vi "Read From VS Parameter FIFO.vi"(8 "Error In":errorcluster, 11 "Async State Vars":T1) -> (0 "Error Out":errorcluster, 1 "Parameter FIFO empty?":bool, 3 "Async State Vars out":T1)   [LabVIEW 2014, in "Waveform-Processing-Custom-Device Engine.lvlib"]
uses:
  Waveform-Processing-Custom-Device Engine.lvlib
  Types/Async State Vars.ctl
  Types/Async FIFOs.ctl
  <vilib>/NI Veristand/Custom Device Waveform API/Single Waveform Read (DBL)/Single Waveform Read (DBL).lvclass
  <vilib>/NI Veristand/Custom Device Waveform API/Single Waveform Write (DBL)/Single Waveform Write (DBL).lvclass
  <vilib>/NI Veristand/Custom Device API/Waveform Data Reference.ctl
  <vilib>/NI Veristand/Custom Device API/Custom Device API.lvlib
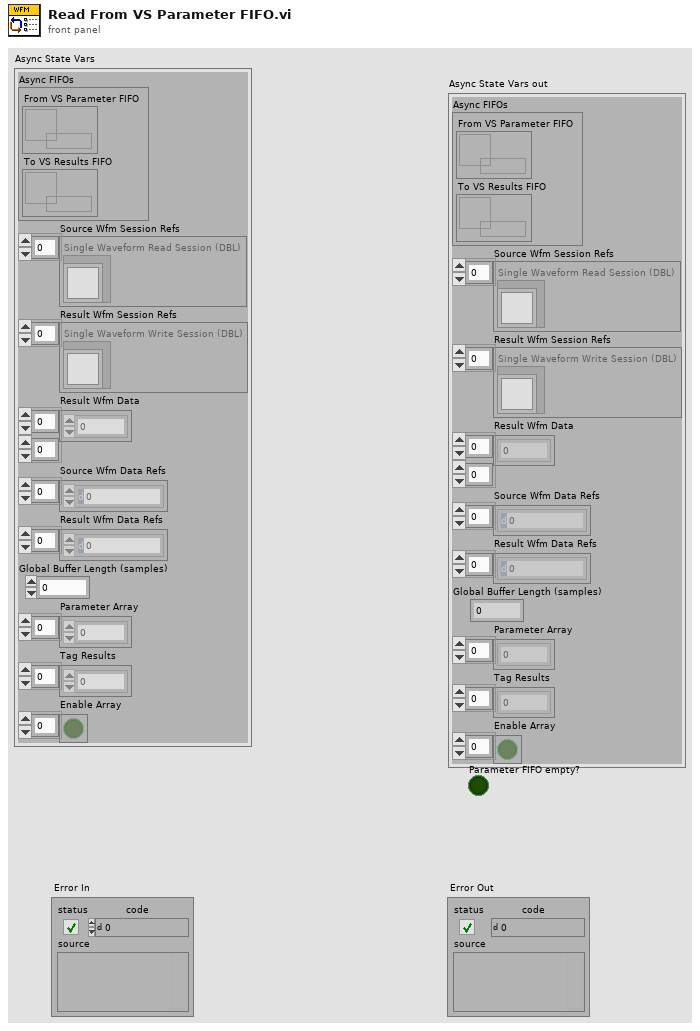
[diagram p1: front panel]
types:
  T1 = typedef "Waveform-Processing-Custom-Device Engine.lvlib/Async State Vars.ctl" = cluster{"Async FIFOs":T2, "Source Wfm Session Refs":refnum<class "Single Waveform Read (DBL).lvclass">[], "Result Wfm Session Refs":refnum<class "Single Waveform Write (DBL).lvclass">[], "Result Wfm Data":dbl[][], "Source Wfm Data Refs":T3[], "Result Wfm Data Refs":T3[], "Global Buffer Length (samples)":dbl, "Parameter Array":dbl[], "Tag Results":dbl[], "Enable Array":bool[]}
  T2 = typedef "Waveform-Processing-Custom-Device Engine.lvlib/Async FIFOs.ctl" = cluster{"From VS Parameter FIFO":refnum<k33>, "To VS Results FIFO":refnum<k33>}
  T3 = typedef "Custom Device API.lvlib/Waveform Data Reference.ctl" = i32
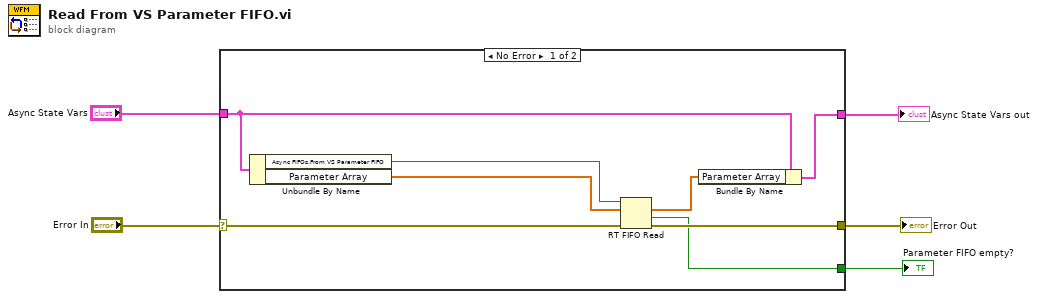
[diagram p0: block diagram]
diagram:
  n1 = case shown="No Error" "Error In" {
    selector: "Error In" -> [w11 w15]
    tunnel: [w8 w15] -> w4
    tunnel: "Async State Vars" -> [w10 w14]
    tunnel: [w7 w14] -> w2
    tunnel: [w6 _] -> w1
    frame No Error {
      n2 = Unbundle By Name(w10) -> ("Async FIFOs.From VS Parameter FIFO"=w13:refnum<k33>, "Parameter Array"=w12:dbl[])
      n3 = RT FIFO Read(0:w13, 1:w12, 3:w11) -> (9:w9:dbl[], 10:w6:bool, 11:w8:errorcluster)  [unwired: 1 in, 2 out]
      n4 = Bundle By Name(cluster=w10, "Parameter Array"=w9) -> (w7:T1)
    }
    frame Error {
    }
  }
  "Error Out" <- w4
  "Async State Vars out" <- w2
  "Parameter FIFO empty?" <- w1
